vi "TranslateVi.vi"(8 "error in (no error)":errorcluster, 11 "VI ref":refnum<vi>) -> (0 "error out":errorcluster)   [LabVIEW 2011]
uses:
  Dictionnary/EnumCommandDictionnaire.ctl
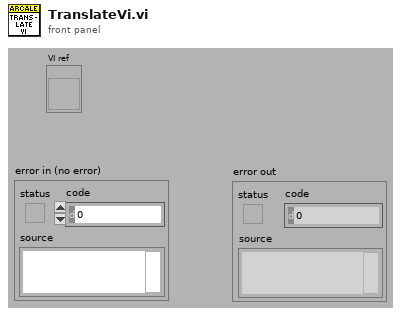
[diagram p1: front panel]
types:
  T1 = typedef "EnumCommandDictionnaire.ctl" = enum16{"Load", "Translate", "Save", "GetDico", "Set : A traduire = Vrai", "Set : A Traduire = Faux", "SetDico"}
  T2 = typedef "Dictionnaire.ctl" = cluster{"FichierDictionnaire":path, "TabCleValeur":T3[], "DictionnaireModifié?":bool, "Traduction à réaliser ?":bool, "Interdire l'ajout de nouvelles clés ?":bool}
  T3 = typedef "CleValeur.ctl" = cluster{"Clé":string, "Valeur":string}
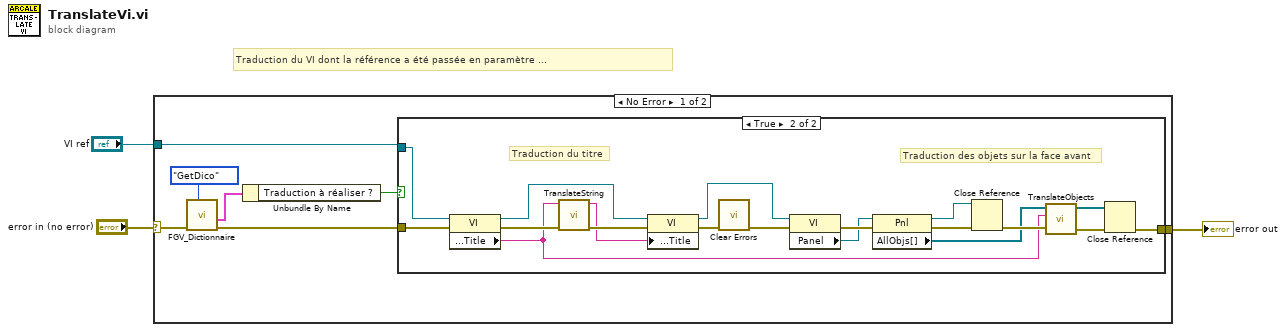
[diagram p0: block diagram]
diagram:
  # "Traduction du VI dont la référence a été passée en paramètre ..."
  n1 = case shown="No Error" "error in (no error)" {
    selector: "error in (no error)" -> [w8 w31]
    tunnel: "VI ref" -> [w10 _]
    tunnel: [w9 w31] -> w1
    frame No Error {
      n2 = call "FGV_Dictionnaire.vi"("Command"=EnumCommandDictionnaire."GetDico", "error in (no error)"=w8) -> ("error out"=w7:errorcluster, "Dictionnaire Out"=w5:T2)  [unwired: 7 in, 1 out]
      n3 = Unbundle By Name(w5) -> ("Traduction à réaliser ?"=w4:bool)
      n4 = case shown="True" w4 {
        tunnel: w10 -> [_ w30]
        tunnel: [w11 w23] -> w9
        tunnel: w7 -> [w11 w22]
        frame False {
        }
        frame True {
          # "Traduction des objets sur la face avant"
          # "Traduction du titre"
          n5 = property class="VI"(reference=w30, error in=w22) -> (reference out=w16:refnum<vi>, error out=w20:errorcluster, "Front Panel.Title"=w18:string)
          n6 = call "TranslateString.vi"("error in (no error)"=w20, "String"=w18) -> ("error out"=w19:errorcluster, "Translated String"=w17:string)  [unwired: 8 in]
          n7 = property class="VI"(reference=w16, error in=w19, "Front Panel.Title"=w17) -> (reference out=w12:refnum<vi>, error out=w21:errorcluster)
          n8 = call <vilib>:"Clear Errors.vi"("error in (no error)"=w21) -> ("error out"=w15:errorcluster)  [unwired: 6 in]
          n9 = property class="VI"(reference=w12, error in=w15) -> (error out=w14:errorcluster, "Panel"=w13:refnum<vi>)  [unwired: 1 out]
          n10 = property class="Pnl"(reference=w13, error in=w14) -> (reference out=w26:refnum<vi>, error out=w28:errorcluster, "AllObjs[]"=w25:refnum<vi>[])
          n11 = Close Reference(reference=w26, error in (no error)=w28) -> (error out=w27:errorcluster)
          n12 = call "TranslateObjects.vi"("errorIN"=w27, "Cle"=w18, "AllObjs[]In"=w25) -> ("error out"=w29:errorcluster, "AllObjs[]Out"=w24:refnum<vi>[])  [unwired: 7 in]
          n13 = Close Reference(reference=w24, error in (no error)=w29) -> (error out=w23:errorcluster)
        }
      }
    }
    frame Error {
    }
  }
  "error out" <- w1
